vi "LakeShore335 Control Panel.vi"(8 "error in (no error)":errorcluster, 11 "LakeShore 335 in":refnum<class "LakeShore 335.lvclass">) -> (0 "error out":errorcluster, 3 "Class":refnum<class "LakeShore 335.lvclass">)   [LabVIEW 2015, in "LakeShore 335.lvclass"]
uses:
  LakeShore 335.lvclass
  LakeShore335 Front Panel Data.ctl
  LakeShore335 Heater Ranges.ctl
  Neocera/Neocera Set Point Aproach.ctl
panel:
  in  "Data":T1={"Heater"=FALSE, "A"=TRUE, "B"=FALSE, " RAW"=FALSE, "Set point"=0.0, "Set Heater Range"=enum."0 (Off)", "Approach"=enum."Instant", "Ramp rate, K/min"=0.0}
  # "Temperature Monitor"
  # "Record Channels"
  # "Temperature Control"
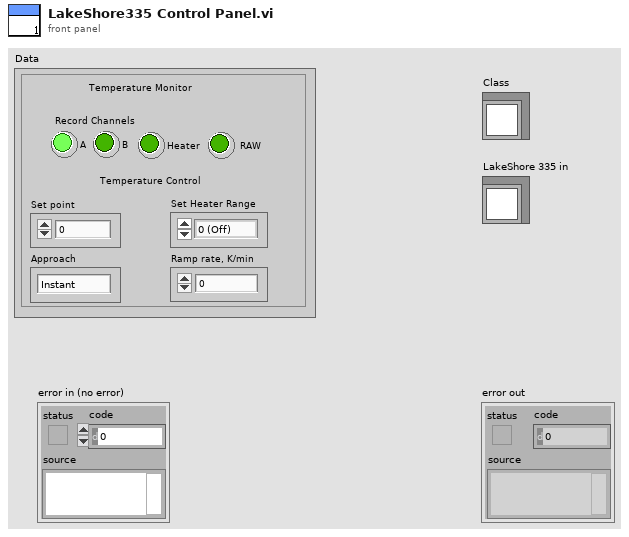
[diagram p1: front panel]
types:
  T1 = typedef "LakeShore335 Front Panel Data.ctl" = cluster{"Heater":bool, "A":bool, "B":bool, " RAW":bool, "Set point":dbl, "Set Heater Range":T2, "Approach":T3, "Ramp rate, K/min":dbl}
  T2 = typedef "LakeShore335 Heater Ranges.ctl" = enum16{"0 (Off)", "1 Low", "2 Medium", "3 High"}
  T3 = typedef "Neocera Set Point Aproach.ctl" = enum16{"Instant", "Ramp"}
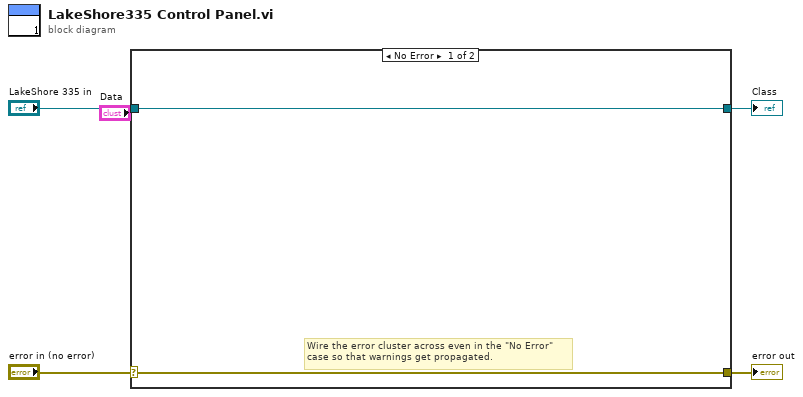
[diagram p0: block diagram]
diagram:
  n1 = case shown="No Error" "error in (no error)" {
    selector: "error in (no error)" -> [w5 w8]
    tunnel: [w5 w8] -> w3
    tunnel: [w6 w7] -> w1
    tunnel: "LakeShore 335 in" -> [w6 w7]
    frame No Error {
      # "Wire the error cluster across even in the \"No Error\"\ncase so that warnings get propagated."
    }
    frame Error {
    }
  }
  "error out" <- w3
  "Class" <- w1
